vi "Write.vi"(8 "error in (no error)":errorcluster, 10 "Write Buffer (\"\")":string, 11 "VISA resource name":refnum<visa-resource-name>) -> (0 "error out":errorcluster, 2 "Return Count":u32, 3 "VISA resource name out":refnum<visa-resource-name>)   [LabVIEW 2009, in "DSO1K.lvlib"]
doc: "Writes the data."
uses:
  <instrlib>/DSO1K/DSO1K.lvlib
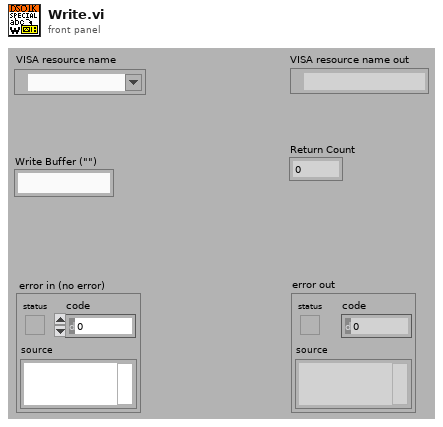
[diagram p1: front panel]
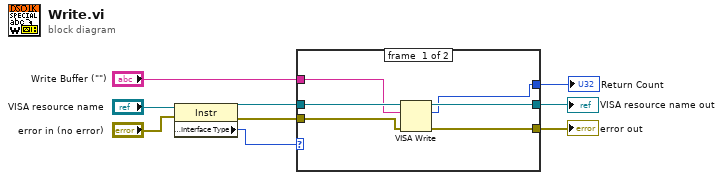
[diagram p0: block diagram]
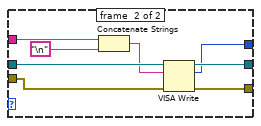
[diagram p2: hidden frame]
diagram:
  n1 = property class="Instr"(reference="VISA resource name", error in="error in (no error)") -> (reference out=w9:refnum<visa-resource-name>, error out=w8:errorcluster, "Interface Information:Interface Type"=w6:u16)
  n2 = case shown="4, 6, Default" w6 {
    tunnel: [w15 w17] -> w4
    tunnel: w9 -> [w14 w22]
    tunnel: [w12 w18] -> w3
    tunnel: w8 -> [w11 w21]
    tunnel: "Write Buffer (\"\")" -> [w13 w23]
    tunnel: [w10 w16] -> w5
    frame #0 {
      n3 = VISA Write(VISA resource name=w14, write buffer=w13, error in (no error)=w11) -> (VISA resource name out=w15:refnum<visa-resource-name>, return count=w10:u32, error out=w12:errorcluster)
    }
    frame #1 {
      n4 = Concatenate Strings(w23, "\n") -> (w19:string)
      n5 = VISA Write(VISA resource name=w22, write buffer=w19, error in (no error)=w21) -> (VISA resource name out=w17:refnum<visa-resource-name>, return count=w16:u32, error out=w18:errorcluster)
    }
  }
  "error out" <- w3
  "VISA resource name out" <- w4
  "Return Count" <- w5
